vi "Dequeue Message.vi"(8 "error in (no error)":errorcluster, 10 "timeout in ms (-1)":i32=-1, 11 "Message Queue":refnum<queue>) -> (0 "error out":errorcluster, 1 "Message Data":variant, 2 "Message":string, 3 "dup Message Queue":refnum<queue>)   [LabVIEW 2020, in "ChromTech Next Gen Compensator Pump.lvlib" / "Message Queue.lvlib"]
doc: "This VI pulls messages off the Message Queue."
uses:
  Message Queue.lvlib
  Message Cluster.ctl
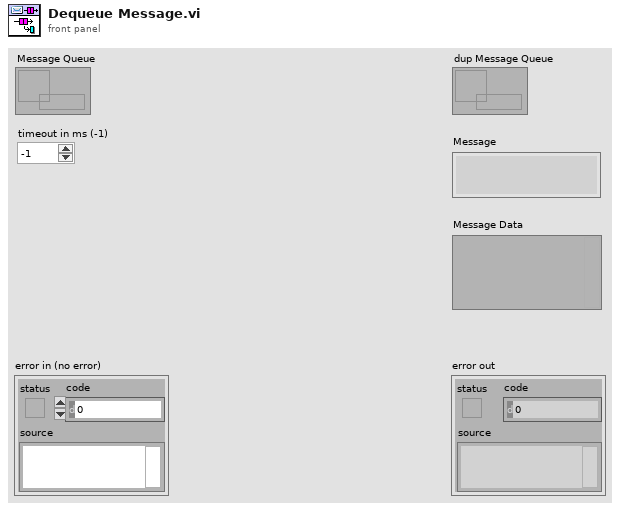
[diagram p1: front panel]
types:
  T1 = typedef "ChromTech Next Gen Compensator Pump.lvlib/Message Queue.lvlib/Message Cluster.ctl" = cluster{"Message":string, "Message Data":variant}
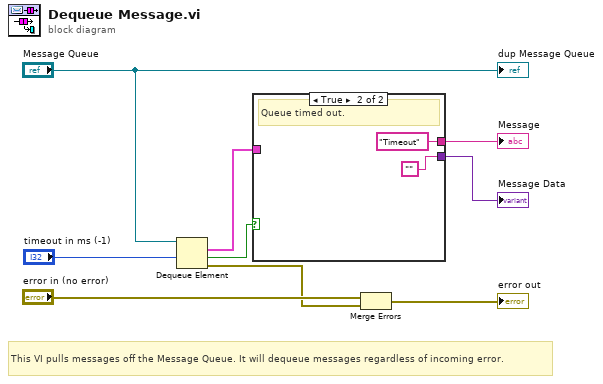
[diagram p0: block diagram]
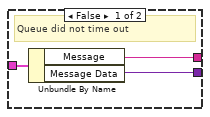
[diagram p2: hidden frame]
diagram:
  # "This VI pulls messages off the Message Queue. It will dequeue messages regardless of incoming error."
  n1 = Dequeue Element(queue="Message Queue", timeout in ms (-1)="timeout in ms (-1)") -> (element=w6:T1, timed out?=w1:bool, error out=w3:errorcluster)  [unwired: 1 in, 1 out]
  n2 = case shown="True" w1 {
    tunnel: [w12 "Timeout" ("Message")] -> w8
    tunnel: [w11 ""] -> w7
    tunnel: w6 -> [w10 _]
    frame False {
      # "Queue did not time out"
      n3 = Unbundle By Name(w10) -> ("Message"=w12:string, "Message Data"=w11:variant)
    }
    frame True {
      # "Queue timed out."
    }
  }
  "Message" <- w8
  "Message Data" <- w7
  n4 = Merge Errors("error in (no error)", w3) -> (→"error out":errorcluster)
  "dup Message Queue" <- "Message Queue"
